vi "final project.vi"() -> ()   [LabVIEW 2020]
panel:
  out "Everything Is Good":bool
  out "Fire":bool
  out "Intruder":bool
  in  "COM Port":refnum<visa-resource-name>
  in  "Table Control":string[][](table)
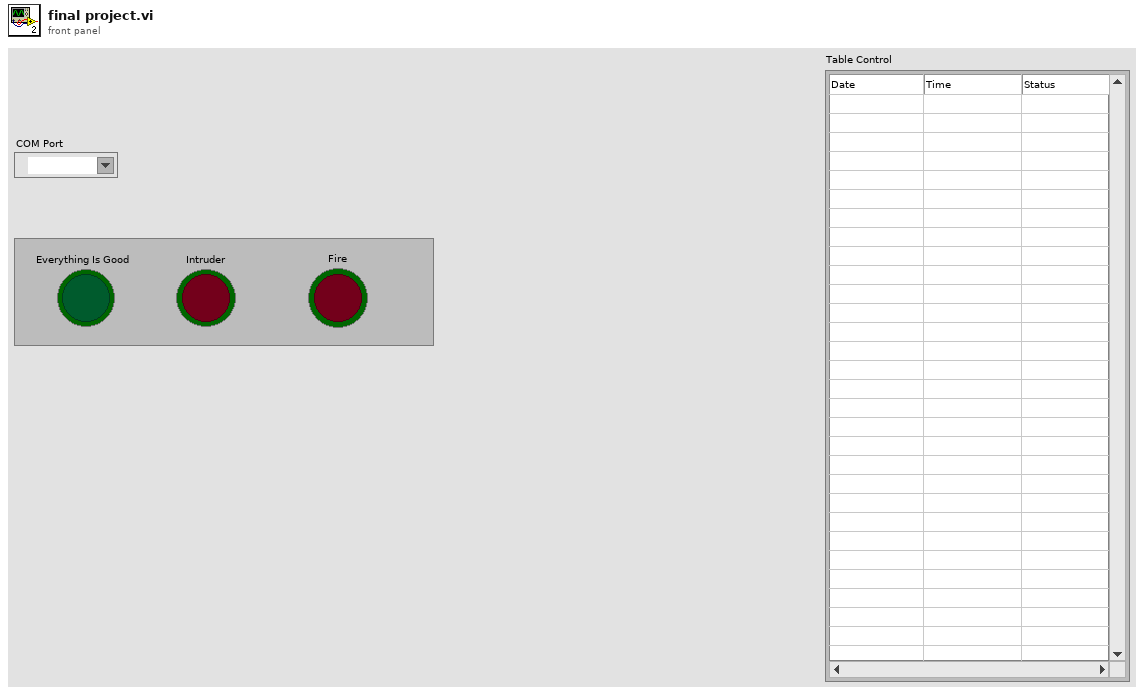
[diagram p1: front panel]
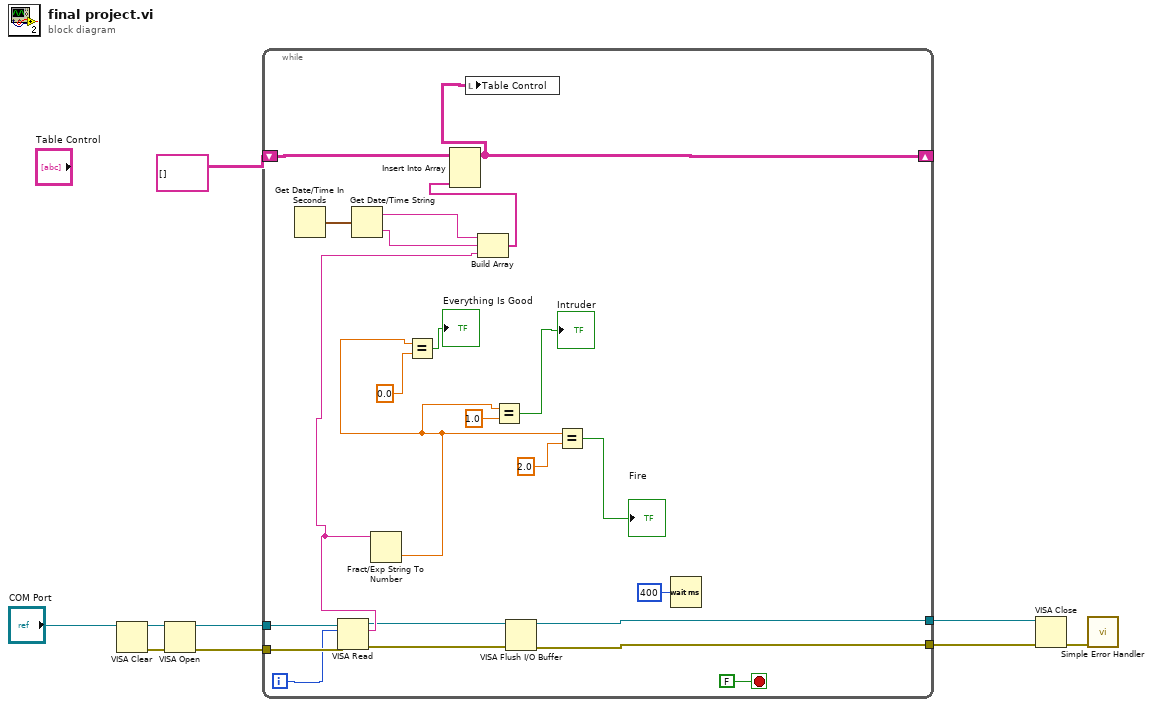
[diagram p0: block diagram]
diagram:
  n1 = VISA Clear(VISA resource name="COM Port") -> (VISA resource name out=w8:refnum<visa-resource-name>, error out=w9:errorcluster)  [unwired: 1 in]
  n2 = VISA Open(error in (no error)=w9, VISA resource name=w8) -> (VISA resource name=w6:refnum<visa-resource-name>, error out=w5:errorcluster)  [unwired: 3 in]
  n3 = while {
    tunnel: w6 -> [w32]
    tunnel: w5 -> [w31]
    tunnel: [w30] -> w4
    tunnel: [w29] -> w3
    shift-right: [w25] -> _
    shift-left: string[][] [] -> [w26]
    i -> [w28]
    stop <- FALSE stop-if-true
    n4 = Get Date/Time In Seconds() -> (seconds since 1Jan1904=w24:timestamp)
    n5 = VISA Read(VISA resource name=w32, byte count=w28, error in (no error)=w31) -> (VISA resource name out=w11:refnum<visa-resource-name>, read buffer=w12:string, error out=w10:errorcluster)  [unwired: 1 out]
    n6 = Get Date/Time String(seconds (now)=w24) -> (date string=w23:string, time string=w22:string)  [unwired: 2 in]
    n7 = Fract/Exp String To Number(string=w12) -> (number=w16:dbl)  [unwired: 3 in, 1 out]
    n8 = Equal?(x=w16, y=0.0) -> (x = y?=→"Everything Is Good":bool)
    n9 = Build Array(w23, w22, w12) -> (w21:string[])
    n10 = Insert Into Array(array=w26, new element=w21) -> (w25:string[][])  [unwired: 2 in]
    n11 = local write "Table Control"(w25) -> ()
    n12 = Equal?(x=w16, y=1.0) -> (x = y?=→"Intruder":bool)
    n13 = VISA Flush I/O Buffer(VISA resource name=w11, error in (no error)=w10) -> (VISA resource name out=w30:refnum<visa-resource-name>, error out=w29:errorcluster)  [unwired: 1 in]
    n14 = Equal?(x=w16, y=2.0) -> (x = y?=→"Fire":bool)
    n15 = Wait (ms)(milliseconds to wait=u32 400) -> ()  [unwired: 1 out]
  }
  n16 = VISA Close(VISA resource name=w4, error in (no error)=w3) -> (error out=w7:errorcluster)
  n17 = call <vilib>:"Simple Error Handler.vi"("error in (no error)"=w7) -> ()  [unwired: 4 in, 5 out]
